vi "Stop Torque Monitor.vi"(0 "reference in":refnum<class "SmartMotor.lvclass">, 5 "error in (no error)":errorcluster) -> (14 "reference out":refnum<class "SmartMotor.lvclass">, 19 "error out":errorcluster)   [LabVIEW 2017, in "SmartMotor.lvclass"]
uses:
  SmartMotor.lvclass
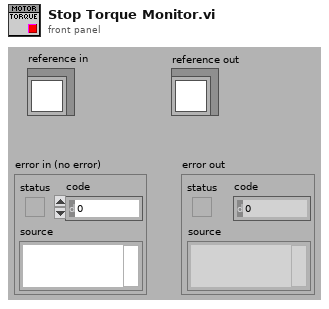
[diagram p1: front panel]
types:
  T1 = typedef "SmartMotor.lvclass/ObjectAttributes.ctl" = cluster{"SmartMotor Chain VISA Resource":refnum<visa-resource-name>, "SmartMotor Chain Address":i16, "Motor Absolute Position":i32, "Motor Relative Position":i32, "Motor Torque":i32, "Motor Voltage":i32, "Screwdriver Engaged":bool, "Screwdriver Torque Limit":i32, "Torque Monitor On/Off Status":bool, "Torque Monitor VI Reference":refnum<vi>, "Absolute Motor Torque (Filtered)":dbl, "SmartMotor Status":T2, "SmartMotor Error":T3}
  T2 = typedef "SmartMotor.lvclass/SmartMotor Status.ctl" = enum8{"Stopped", "Moving"}
  T3 = typedef "SmartMotor.lvclass/SmartMotor Error.ctl" = enum8{"None", "Read Error", "Low Voltage"}
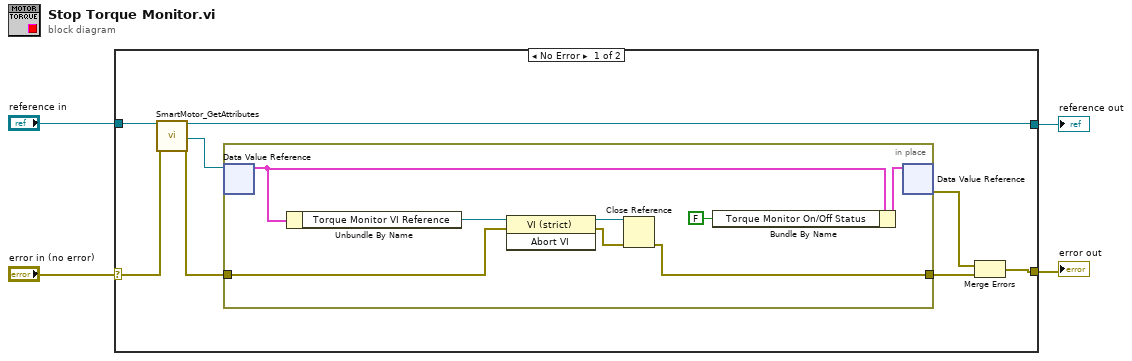
[diagram p0: block diagram]
diagram:
  n1 = case shown="No Error" "error in (no error)" {
    selector: "error in (no error)" -> [w11 w22]
    tunnel: [w8 w22] -> w3
    tunnel: [w9 w21] -> w1
    tunnel: "reference in" -> [w12 w21]
    frame No Error {
      n2 = call "SmartMotor_GetAttributes.vi"("reference in"=w12, "error in (no error)"=w11) -> ("reference out"=w9:refnum<class "SmartMotor.lvclass">, "DataRef"=w7:refnum<data-value>, "error out"=w6:errorcluster)  [unwired: 14 in, 1 out]
      n3 = in-place {
        in-place-border: w6 -> [w15]
        in-place-border: [w13] -> w5
        n4 = in-place-dvr #1(w7) -> (w19:T1)  [unwired: 1 out]
        n5 = Unbundle By Name(w19) -> ("Torque Monitor VI Reference"=w17:refnum<vi>)
        n6 = invoke class="VI (strict)" method="Abort VI"(reference=w17, error in=w15) -> (reference out=w16:refnum<vi>, error out=w14:errorcluster)  [unwired: 1 in, 1 out]
        n7 = Close Reference(reference=w16, error in (no error)=w14) -> (error out=w13:errorcluster)
        n8 = Bundle By Name(cluster=w19, "Torque Monitor On/Off Status"=FALSE) -> (w20:T1)
        n9 = in-place-dvr #1(w20) -> (w10:errorcluster)  [unwired: 1 out]
      }
      n10 = Merge Errors(w10, w5) -> (w8:errorcluster)
    }
    frame Error {
    }
  }
  "error out" <- w3
  "reference out" <- w1
